vi "Motor Controller Read Live Config or EEPROM.vi"(0 "COM port":refnum<visa-resource-name>, 5 "RS-485 addr.":u8, 7 "Cmd":string(combo)="G", 11 "Close port after action":bool) -> (4 "COM port out":refnum<visa-resource-name>, 6 "EEPROM":T1={"N bits"=8, "dt (s)"=0.0, "Kp (/rpm)"=0.0, "Ti (s)"=0.0, "Td (s)"=0.0, "N bits_soft"=8, "dt_soft (s)"=0.0, "Kp_soft (/rpm)"=0.0, "Ti_soft (s)"=0.0, "Td_soft (s)"=0.0, "Encoder counting edges"=0, "Encoder PPR"=0, "Final drive ratio (X:1)"=0.0, "Current zero offset (A)"=0.0, "RS-485 address"=0, "RS-485 baud rate"=0, "Data output period (us)"=0, "RPM setpoint"=0.0, "USB streaming enabled"=FALSE, "Operating mode"=0, "Running mode"=0, "EEPROM CRC-16"=0} {"Running mode" items=["NORMAL", "SOFT"]; "Operating mode" items=["RUN", "COAST", "BRAKE", "SLEEP"]; "EEPROM CRC-16" format="%04x"; "N bits_soft" min=8 max=16 step=1; "Td_soft (s)" format="%#_6f"; "Ti_soft (s)" format="%#_6f"; "Kp_soft (/rpm)" format="%#_6f"; "dt_soft (s)" format="%#_6f"; "N bits" min=8 max=16 step=1; "Td (s)" format="%#_6f"; "Ti (s)" format="%#_6f"; "Kp (/rpm)" format="%#_6f"; "dt (s)" format="%#_6f"}, 8 "CRC-16 ok":bool, 15 "Error out":errorcluster)   [LabVIEW 2020]
uses:
  ctls/CTRL_EEPROM.ctl
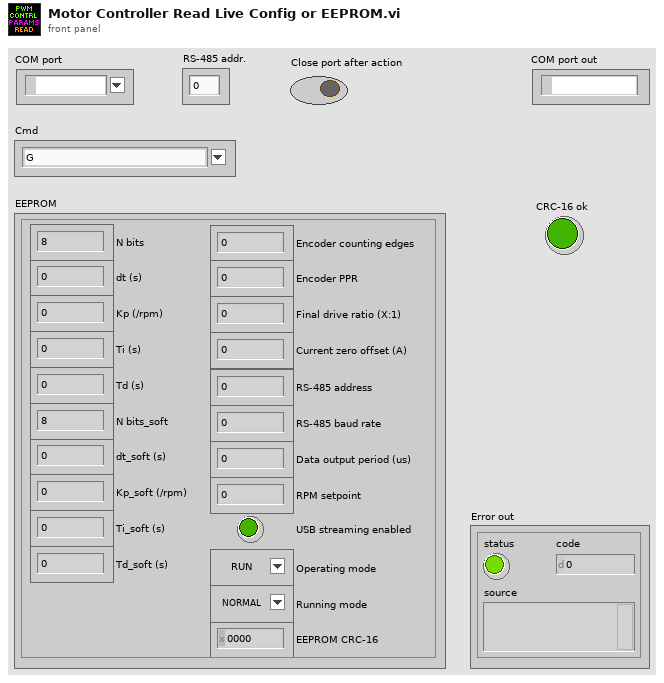
[diagram p1: front panel]
types:
  T1 = typedef "CTRL_EEPROM.ctl" = cluster{"N bits":u8, "dt (s)":sgl, "Kp (/rpm)":sgl, "Ti (s)":sgl, "Td (s)":sgl, "N bits_soft":u8, "dt_soft (s)":sgl, "Kp_soft (/rpm)":sgl, "Ti_soft (s)":sgl, "Td_soft (s)":sgl, "Encoder counting edges":u8, "Encoder PPR":u16, "Final drive ratio (X:1)":sgl, "Current zero offset (A)":sgl, "RS-485 address":u8, "RS-485 baud rate":u32, "Data output period (us)":u32, "RPM setpoint":sgl, "USB streaming enabled":bool, "Operating mode":u8, "Running mode":u8, "EEPROM CRC-16":u16}
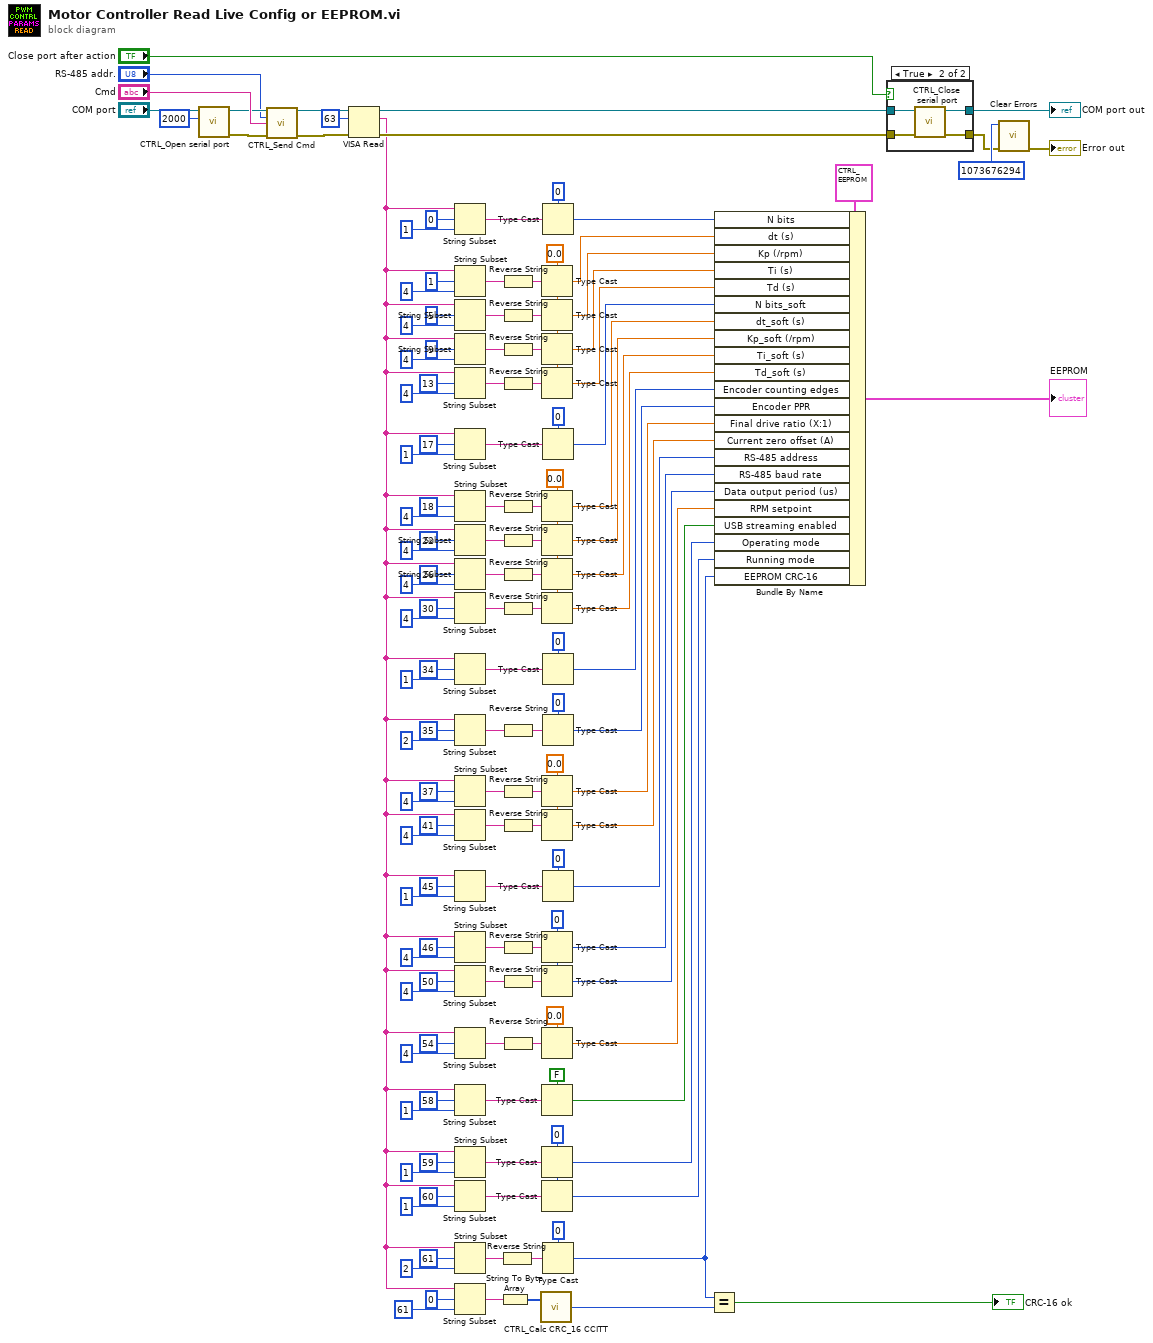
[diagram p0: block diagram]
diagram:
  w9 = u8 0 ("offset (0)")
  w65 = u32 0 ("offset (0)")
  w70 = sgl 0.0 ("offset (0)")
  w107 = sgl 0.0 ("offset (0)")
  w108 = sgl 0.0 ("offset (0)")
  n1 = call "CTRL_Open serial port.vi"("timeout (ms)"=u32 2000, "VISA resource name"="COM port") -> ("Error out"=w136:errorcluster, "VISA resource name out"=w6:refnum<visa-resource-name>)  [unwired: 8 in]
  n2 = call "CTRL_Send Cmd.vi"("Port"=w6, "RS-485 addr."="RS-485 addr.", "Cmd"="Cmd", "Error In"=w136) -> ("Port out"=w134:refnum<visa-resource-name>, "Error Out"=w135:errorcluster)  [unwired: 10 in]
  n3 = VISA Read(VISA resource name=w134, byte count=u32 63, error in (no error)=w135) -> (VISA resource name out=w133:refnum<visa-resource-name>, read buffer=w10:string, error out=w132:errorcluster)  [unwired: 1 out]
  n4 = String Subset(string=w10, offset (0)=0, length (rest)=1 ("length (rest)")) -> (substring=w122:string)
  n5 = String Subset(string=w10, offset (0)=1, length (rest)=4 ("length (rest)")) -> (substring=w112:string)
  n6 = String Subset(string=w10, offset (0)=5, length (rest)=4 ("length (rest)")) -> (substring=w111:string)
  n7 = String Subset(string=w10, offset (0)=9, length (rest)=4 ("length (rest)")) -> (substring=w110:string)
  n8 = String Subset(string=w10, offset (0)=13, length (rest)=4 ("length (rest)")) -> (substring=w109:string)
  n9 = String Subset(string=w10, offset (0)=17, length (rest)=1 ("length (rest)")) -> (substring=w93:string)
  n10 = String Subset(string=w10, offset (0)=18, length (rest)=4 ("length (rest)")) -> (substring=w103:string)
  n11 = String Subset(string=w10, offset (0)=22, length (rest)=4 ("length (rest)")) -> (substring=w104:string)
  n12 = String Subset(string=w10, offset (0)=26, length (rest)=4 ("length (rest)")) -> (substring=w105:string)
  n13 = String Subset(string=w10, offset (0)=30, length (rest)=4 ("length (rest)")) -> (substring=w106:string)
  n14 = String Subset(string=w10, offset (0)=34, length (rest)=1 ("length (rest)")) -> (substring=w84:string)
  n15 = String Subset(string=w10, offset (0)=35, length (rest)=2 ("length (rest)")) -> (substring=w81:string)
  n16 = String Subset(string=w10, offset (0)=37, length (rest)=4 ("length (rest)")) -> (substring=w72:string)
  n17 = String Subset(string=w10, offset (0)=41, length (rest)=4 ("length (rest)")) -> (substring=w71:string)
  n18 = String Subset(string=w10, offset (0)=45, length (rest)=1 ("length (rest)")) -> (substring=w67:string)
  n19 = String Subset(string=w10, offset (0)=46, length (rest)=4 ("length (rest)")) -> (substring=w63:string)
  n20 = String Subset(string=w10, offset (0)=50, length (rest)=4 ("length (rest)")) -> (substring=w64:string)
  n21 = String Subset(string=w10, offset (0)=54, length (rest)=4 ("length (rest)")) -> (substring=w27:string)
  n22 = String Subset(string=w10, offset (0)=58, length (rest)=1 ("length (rest)")) -> (substring=w20:string)
  n23 = String Subset(string=w10, offset (0)=59, length (rest)=1 ("length (rest)")) -> (substring=w14:string)
  n24 = String Subset(string=w10, offset (0)=60, length (rest)=1 ("length (rest)")) -> (substring=w13:string)
  n25 = String Subset(string=w10, offset (0)=61, length (rest)=2 ("length (rest)")) -> (substring=w54:string)
  n26 = String Subset(string=w10, offset (0)=0, length (rest)=61 ("length (rest)")) -> (substring=w33:string)
  n27 = String To Byte Array(string=w33) -> (unsigned byte array=w138:u8[])
  n28 = Reverse String(1:w54) -> (0:w19:string)
  n29 = Reverse String(1:w112) -> (0:w128:string)
  n30 = Reverse String(1:w111) -> (0:w127:string)
  n31 = Reverse String(1:w110) -> (0:w126:string)
  n32 = Reverse String(1:w109) -> (0:w125:string)
  n33 = Reverse String(1:w103) -> (0:w87:string)
  n34 = Reverse String(1:w104) -> (0:w88:string)
  n35 = Reverse String(1:w105) -> (0:w89:string)
  n36 = Reverse String(1:w106) -> (0:w90:string)
  n37 = Reverse String(1:w81) -> (0:w18:string)
  n38 = Reverse String(1:w72) -> (0:w78:string)
  n39 = Reverse String(1:w71) -> (0:w77:string)
  n40 = Reverse String(1:w63) -> (0:w57:string)
  n41 = Reverse String(1:w64) -> (0:w58:string)
  n42 = Reverse String(1:w27) -> (0:w30:string)
  n43 = call "CTRL_Calc CRC_16 CCITT.vi"("Data bytes"=w138) -> ("CRC_16-CCITT"=w32:u16)  [unwired: 1 in]
  n44 = Type Cast(type=w108, x=w128) -> (*(type *) &x=w51:sgl)
  n45 = Type Cast(type=w108, x=w127) -> (*(type *) &x=w50:sgl)
  n46 = Type Cast(type=w108, x=w126) -> (*(type *) &x=w49:sgl)
  n47 = Type Cast(type=w108, x=w125) -> (*(type *) &x=w48:sgl)
  n48 = Type Cast(type=w107, x=w87) -> (*(type *) &x=w46:sgl)
  n49 = Type Cast(type=w107, x=w88) -> (*(type *) &x=w45:sgl)
  n50 = Type Cast(type=w107, x=w89) -> (*(type *) &x=w44:sgl)
  n51 = Type Cast(type=w107, x=w90) -> (*(type *) &x=w43:sgl)
  n52 = Type Cast(type=w70, x=w78) -> (*(type *) &x=w40:sgl)
  n53 = Type Cast(type=w70, x=w77) -> (*(type *) &x=w39:sgl)
  n54 = Type Cast(type=w65, x=w57) -> (*(type *) &x=w37:u32)
  n55 = Type Cast(type=w65, x=w58) -> (*(type *) &x=w36:u32)
  n56 = Type Cast(type=sgl 0.0 ("offset (0)"), x=w30) -> (*(type *) &x=w25:sgl)
  n57 = Type Cast(type=FALSE, x=w20) -> (*(type *) &x=w21:bool)
  n58 = Type Cast(type=w9, x=w14) -> (*(type *) &x=w8:u8)
  n59 = Type Cast(type=w9, x=w13) -> (*(type *) &x=w7:u8)
  n60 = Type Cast(type=u8 0 ("offset (0)"), x=w122) -> (*(type *) &x=w52:u8)
  n61 = Type Cast(type=u8 0 ("offset (0)"), x=w93) -> (*(type *) &x=w47:u8)
  n62 = Type Cast(type=u8 0 ("offset (0)"), x=w84) -> (*(type *) &x=w42:u8)
  n63 = Type Cast(type=u16 0 ("offset (0)"), x=w18) -> (*(type *) &x=w41:u16)
  n64 = Type Cast(type=u8 0 ("offset (0)"), x=w67) -> (*(type *) &x=w38:u8)
  n65 = Type Cast(type=u16 0 ("offset (0)"), x=w19) -> (*(type *) &x=w17:u16)
  n66 = Equal?(x=w17, y=w32) -> (x = y?=→"CRC-16 ok":bool)
  n67 = Bundle By Name(cluster=T1 {"N bits"=8, "dt (s)"=0.0, "Kp (/rpm)"=0.0, "Ti (s)"=0.0, "Td (s)"=0.0, "N bits_soft"=8, "dt_soft (s)"=0.0, "Kp_soft (/rpm)"=0.0, "Ti_soft (s)"=0.0, "Td_soft (s)"=0.0, "Encoder counting edges"=0, "Encoder PPR"=0, "Final drive ratio (X:1)"=0.0, "Current zero offset (A)"=0.0, "RS-485 address"=0, "RS-485 baud rate"=0, "Data output period (us)"=0, "RPM setpoint"=0.0, "USB streaming enabled"=FALSE, "Operating mode"=0, "Running mode"=0, "EEPROM CRC-16"=0} ("EEPROM"), "N bits"=w52, "dt (s)"=w51, "Kp (/rpm)"=w50, "Ti (s)"=w49, "Td (s)"=w48, "N bits_soft"=w47, "dt_soft (s)"=w46, "Kp_soft (/rpm)"=w45, "Ti_soft (s)"=w44, "Td_soft (s)"=w43, "Encoder counting edges"=w42, "Encoder PPR"=w41, "Final drive ratio (X:1)"=w40, "Current zero offset (A)"=w39, "RS-485 address"=w38, "RS-485 baud rate"=w37, "Data output period (us)"=w36, "RPM setpoint"=w25, "USB streaming enabled"=w21, "Operating mode"=w8, "Running mode"=w7, "EEPROM CRC-16"=w17) -> (→"EEPROM":T1)
  n68 = case shown="True" "Close port after action" {
    tunnel: [w143 w146] -> w2
    tunnel: w133 -> [w142 w144]
    tunnel: w132 -> [w143 w145]
    tunnel: [w142 w144] -> w4
    frame False {
    }
    frame True {
      n69 = call "CTRL_Close serial port.vi"("Error in"=w145, "VISA resource name"=w144) -> ("Error out"=w146:errorcluster)  [unwired: 9 in]
    }
  }
  "COM port out" <- w4
  n70 = call <vilib>:"Clear Errors.vi"("error in (no error)"=w2, "specific error code to clear (0: all)"=1073676294) -> ("error out"=→"Error out":errorcluster)  [unwired: 4 in, 1 out]
